vi "tm_setoutputtrigger_40.vi"(6 "Port":i32=1, 8 "error in (no error)":errorcluster, 9 "Programmable Options":cluster{"Width":dbl, "Delay":dbl, "Source":u32}={"Width"=0.003, "Delay"=0.0, "Source"=2} {"Source" items=["Exposure"=1, "Readout End"=2, "V Sync"=3, "H Sync"=4, "Trigger"=6]}, 10 "Type":cluster{"Mode":u32, "Polarity":u32}={"Mode"=1, "Polarity"=1} {"Polarity" items=["Negative"=1, "Positive"=2]; "Mode" items=["Low"=1, "Global Exposure"=2, "Programmable"=3, "Trigger Ready"=4, "High"=5]}, 11 "Handle in":u32) -> (0 "error out":errorcluster, 3 "Handle out":u32)   [LabVIEW 2023]
uses:
  tmcamcon.dll
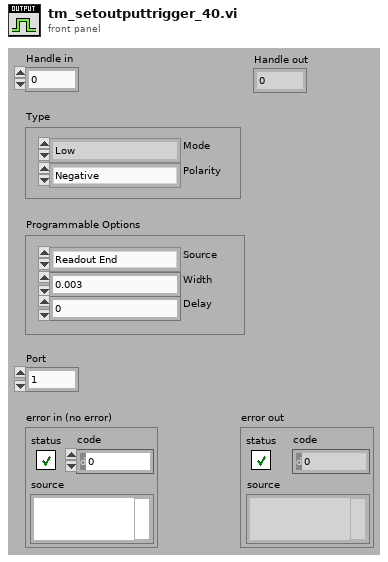
[diagram p1: front panel]
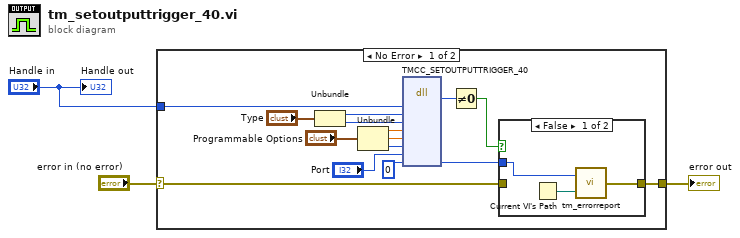
[diagram p0: block diagram]
diagram:
  n1 = case shown="No Error" "error in (no error)" {
    selector: "error in (no error)" -> [w14 w23]
    tunnel: [w11 w23] -> w2
    tunnel: "Handle in" -> [w15 _]
    frame No Error {
      n2 = Unbundle("Type") -> ("Mode"=w9:u32, "Polarity"=w8:u32)
      n3 = Unbundle("Programmable Options") -> ("Width"=w6:dbl, "Delay"=w5:dbl, "Source"=w4:u32)
      n4 = dll-call lib="tmcamcon.dll" fn="TMCC_SETOUTPUTTRIGGER_40"("HDCAM"=w15, "mode"=w9, "polarity"=w8, "period"=w6, "delay"=w5, "source"=w4, "index"="Port", "Erval"=0) -> ("return type"=w18:u32, "Erval"=w13:i32)  [unwired: 10 in, 2 out]
      n5 = Not Equal To 0?(x=w18) -> (x != 0?=w12:bool)
      n6 = case shown="False" w12 {
        tunnel: w14 -> [_ w22]
        tunnel: [w20 w22] -> w11
        tunnel: w13 -> [w19 _]
        frame False {
          n7 = Current VI's Path() -> (path=w21:path)
          n8 = call "tm_errorreport.vi"("Source"=w21, "Error"=w19) -> ("error out"=w20:errorcluster)
        }
        frame True {
        }
      }
    }
    frame Error {
    }
  }
  "error out" <- w2
  "Handle out" <- "Handle in"
